vi "CalcZoomFactor.vi"(8 "error in (no error)":errorcluster, 10 "Image Array":T2[](array[typedef]), 11 "Pict Refnum":refnum<vi>) -> (0 "error out":errorcluster, 2 "ZoomFactor":dbl, 3 "OriginPoint":T1)   [LabVIEW 2019, in "AnimatorXControl.xctl"]
uses:
  AnimatorXControl.xctl
  <vilib>/picture/picture.llb/imagedata.ctl
  <vilib>/Utility/miscctls.llb/LVPointTypeDef.ctl
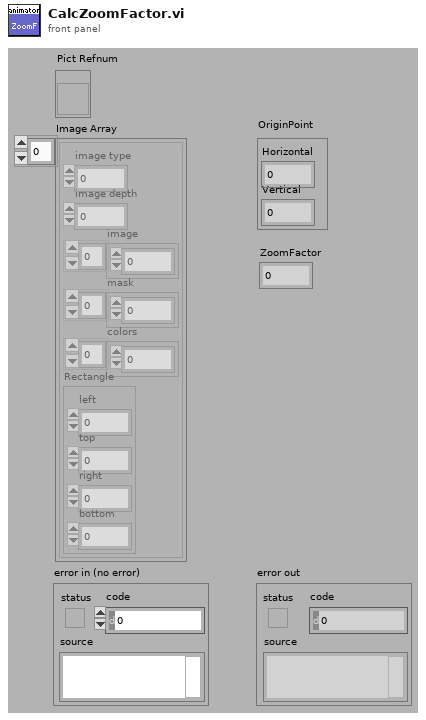
[diagram p1: front panel]
types:
  T1 = typedef "LVPointTypeDef.ctl" = cluster{"Horizontal":i16, "Vertical":i16}
  T2 = typedef "imagedata.ctl" = cluster{"image type":i32, "image depth":i32, "image":u8[], "mask":u8[], "colors":u32[], "Rectangle":cluster{"left":i16, "top":i16, "right":i16, "bottom":i16}}
  T3 = typedef "LVBoundsTypeDef.ctl" = cluster{"Width":u32, "Height":u32}
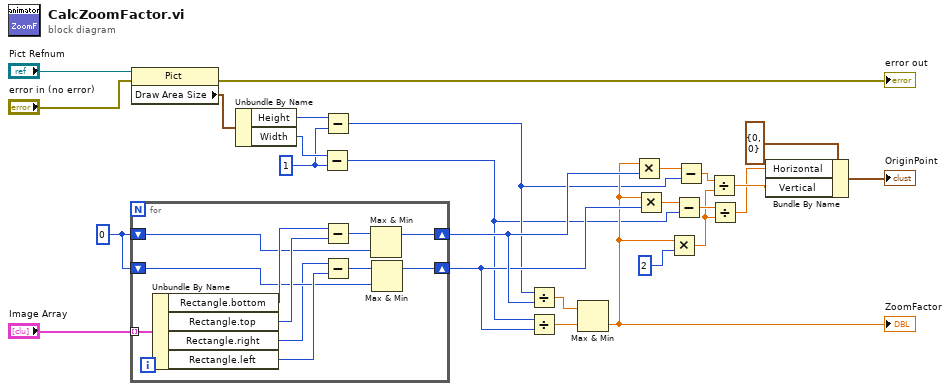
[diagram p0: block diagram]
diagram:
  w4 = u32 1 ("y")
  w26 = u32 0
  n1 = for {
    tunnel: "Image Array" -> [w37] mode=indexing
    shift-right: [w28] -> w22
    shift-left: w26 -> [w32]
    shift-right: [w27] -> w16
    shift-left: w26 -> [w30]
    n2 = Unbundle By Name(w37) -> ("Rectangle.bottom"=w36:i16, "Rectangle.top"=w35:i16, "Rectangle.right"=w29:i16, "Rectangle.left"=w34:i16)
    n3 = Subtract(x=w36, y=w35) -> (x-y=w33:i16)
    n4 = Subtract(x=w29, y=w34) -> (x-y=w31:i16)
    n5 = Max & Min(x=w33, y=w32) -> (max(x,y)=w28:u32)  [unwired: 1 out]
    n6 = Max & Min(x=w31, y=w30) -> (max(x,y)=w27:u32)  [unwired: 1 out]
  }
  n7 = property class="Pict"(reference="Pict Refnum", error in="error in (no error)") -> (error out=→"error out":errorcluster, "Draw Area Size"=w3:T3)  [unwired: 1 out]
  n8 = Unbundle By Name(w3) -> ("Height"=w6:u32, "Width"=w5:u32)
  n9 = Subtract(x=w5, y=w4) -> (x-y=w1:u32)
  n10 = Subtract(x=w6, y=w4) -> (x-y=w2:u32)
  n11 = Divide(x=w2, y=w22) -> (x/y=w25:dbl)
  n12 = Divide(x=w1, y=w16) -> (x/y=w24:dbl)
  n13 = Max & Min(x=w25, y=w24) -> (min(x,y)=w7:dbl)  [unwired: 1 out]
  "ZoomFactor" <- w7
  n14 = Multiply(x=w7, y=w22) -> (x*y=w23:dbl)
  n15 = Multiply(x=w7, y=w16) -> (x*y=w21:dbl)
  n16 = Multiply(x=w7, y=2) -> (x*y=w17:dbl)
  n17 = Subtract(x=w21, y=w1) -> (x-y=w19:dbl)
  n18 = Subtract(x=w23, y=w2) -> (x-y=w20:dbl)
  n19 = Divide(x=w20, y=w17) -> (x/y=w15:dbl)
  n20 = Divide(x=w19, y=w17) -> (x/y=w14:dbl)
  n21 = Bundle By Name(cluster=T1 {"Horizontal"=0, "Vertical"=0} ("Origin"), "Horizontal"=w14, "Vertical"=w15) -> (→"OriginPoint":T1)
